vi "CreateReaderFromLib.vi"(0 "LibPath/LvLibRef":variant, 5 "error in":errorcluster) -> (14 "LibReader out":refnum<class "LibReader.lvclass">, 15 "Description":string, 16 "DataFlowClass":bool, 19 "error out":errorcluster)   [LabVIEW 2014, in "LibReader.lvclass"]
uses:
  <resource>/Framework/Providers/Open_GDS/ClassProviders/LibProvider_BaseClassInterface/LibReader_class/LibReader.lvclass
  <resource>/Framework/Providers/Open_GDS/ClassProviders/Provider_LvNativeClass/ClassReaderNative_class/ClassReaderNative.lvclass
  <resource>/Framework/Providers/Open_GDS/ClassProviders/Provider_EndevoGOOP300/ClassReaderGOOP300_class/ClassReaderGOOP300.lvclass
  <resource>/Framework/Providers/Open_GDS/ClassProviders/Provider_EndevoGOOP400/ClassReaderGOOP400_class/ClassReaderGOOP400.lvclass
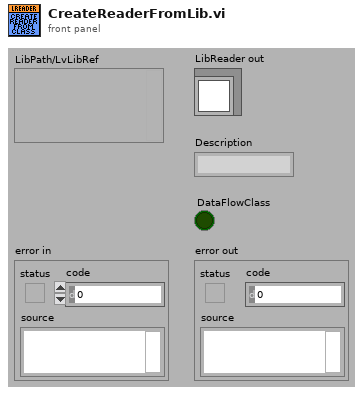
[diagram p1: front panel]
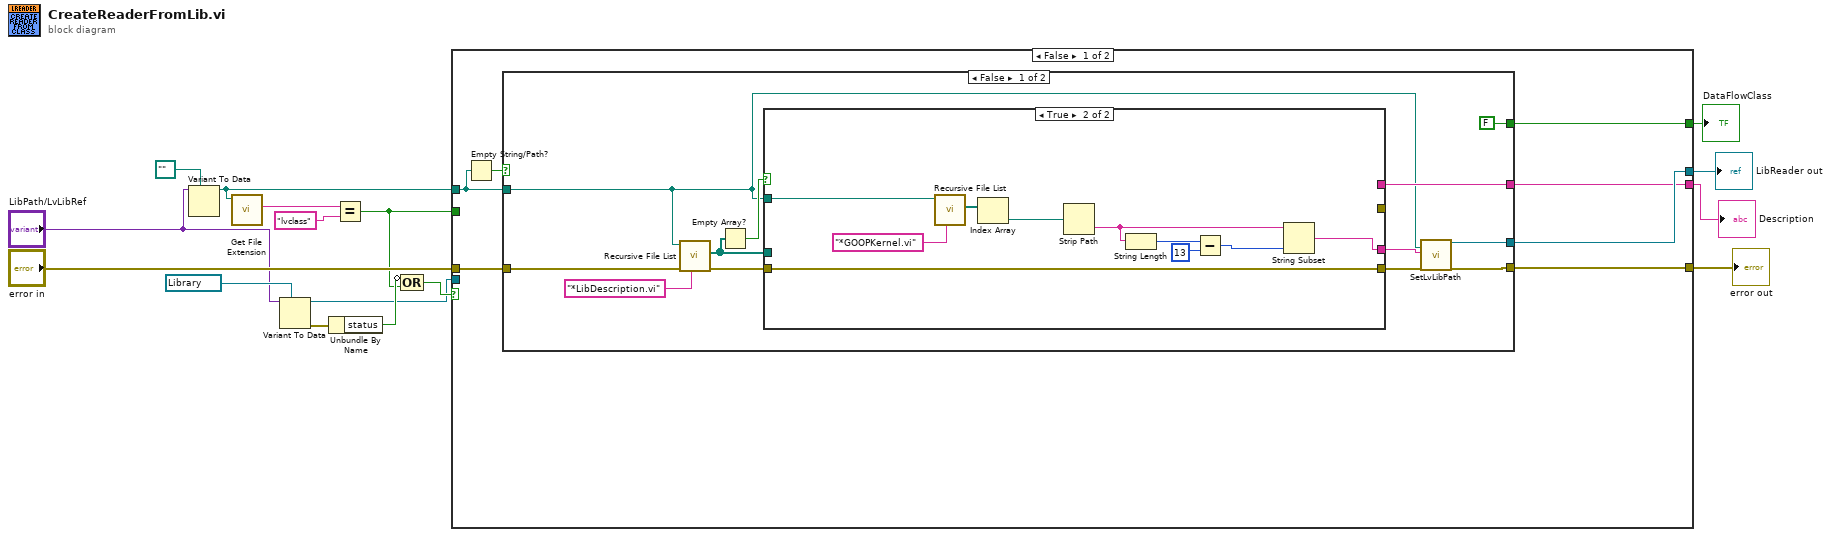
[diagram p0: block diagram]
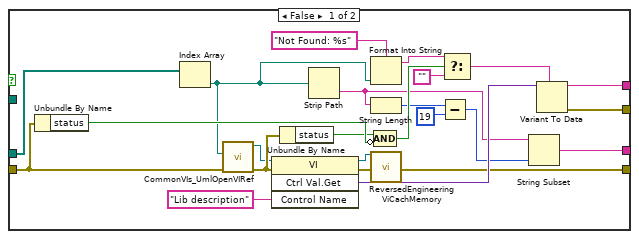
[diagram p2: hidden frame]
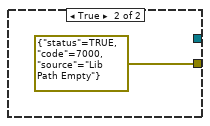
[diagram p3: hidden frame]
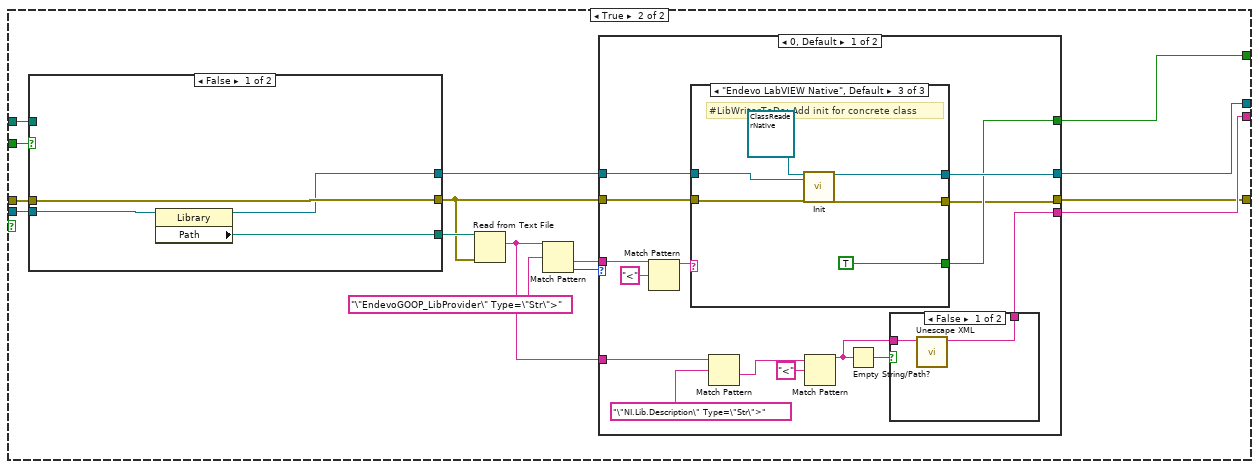
[diagram p4: hidden frame]
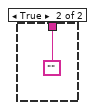
[diagram p5: hidden frame]
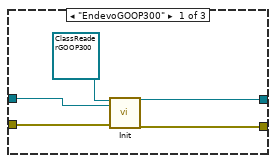
[diagram p6: hidden frame]
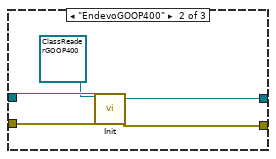
[diagram p7: hidden frame]
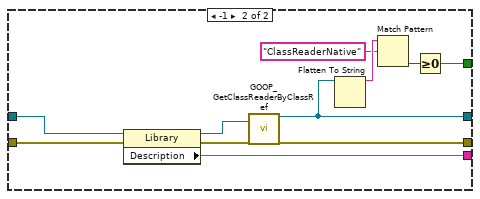
[diagram p8: hidden frame]
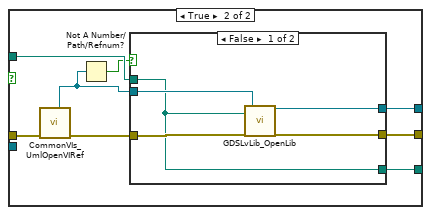
[diagram p9: hidden frame]
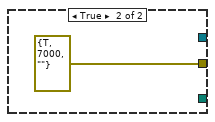
[diagram p10: hidden frame]
diagram:
  n1 = Variant To Data(type=path "", Variant="LibPath/LvLibRef") -> (data=w4:path)  [unwired: 1 in, 1 out]
  n2 = call <vilib>:"Get File Extension.vi"("file"=w4) -> ("lowercase file extension"=w9:string)  [unwired: 7 in, 3 out]
  n3 = Variant To Data(type=refnum<vi> refnum ("LVClass.Open"), Variant="LibPath/LvLibRef") -> (data=w3:refnum<vi>, error out=w7:errorcluster)  [unwired: 1 in]
  n4 = Unbundle By Name(w7) -> ("status"=w6:bool)
  n5 = Equal?(x=w9, y="lvclass") -> (x = y?=w2:bool)
  n6 = Compound Arithmetic op=OR(invert w6, w2) -> (w5:bool)
  n7 = case shown="False" w5 {
    tunnel: [w21 w85] -> w16
    tunnel: "error in" -> [w20 w83]
    tunnel: [w23 w78] -> w14
    tunnel: [w22 w82] -> w13
    tunnel: w4 -> [w18 w81]
    tunnel: w3 -> [_ w79]
    tunnel: w2 -> [_ w80]
    tunnel: [w19 w71] -> w1
    frame False {
      n8 = Empty String/Path?(string/path=w18) -> (empty?=w17:bool)
      n9 = case shown="False" w17 {
        tunnel: [w35 _] -> w23
        tunnel: [w34 errorcluster {"status"=TRUE, "code"=7000, "source"="Lib Path Empty"} ("error out")] -> w22
        tunnel: [w33 _] -> w21
        tunnel: w20 -> [w29 _]
        tunnel: [FALSE _] -> w19
        tunnel: w18 -> [w24 _]
        frame False {
          n10 = call <vilib>:"Recursive File List.vi"("pattern"="*LibDescription.vi" ("FileSearchPattern"), "error in (no error)"=w29, "Folder Path"=w24) -> ("error out"=w28:errorcluster, "All Files in Dir"=w26:path[])  [unwired: 4 in, 3 out]
          n11 = Empty Array?(array=w26) -> (empty?=w31:bool)
          n12 = case shown="True" w31 {
            tunnel: w28 -> [w45 w69]
            tunnel: [w50 _] -> w33
            tunnel: [w47 w69] -> w32
            tunnel: w26 -> [w46 _]
            tunnel: [w37 w60] -> w30
            tunnel: w24 -> [_ w68]
            tunnel: [w36 _] -> _
            frame False {
              n13 = Unbundle By Name(w45) -> ("status"=w52:bool)
              n14 = Index Array(array=w46) -> (element=w42:path)  [unwired: 1 in]
              n15 = call <resource>:"CommonVIs_UmlOpenVIRef.vi"("error in"=w45, "ViPath/ViName"=w42) -> ("error out"=w44:errorcluster, "vi reference"=w43:refnum<vi>)  [unwired: 6 in, 2 out]
              n16 = invoke class="VI" method="Ctrl Val.Get"(reference=w43, error in=w44, "Control Name"="Lib description") -> (reference out=w59:refnum<vi>, error out=w48:errorcluster, "Get Control Value Variant"=w58:variant)  [unwired: 1 in, 1 out]
              n17 = Unbundle By Name(w44) -> ("status"=w51:bool)
              n18 = Strip Path(path=w42) -> (name=w41:string)  [unwired: 1 out]
              n19 = Format Into String(format string="Not Found: %s", w42) -> (resulting string=w56:string)  [unwired: 2 in, 1 out]
              n20 = String Length(string=w41) -> (length=w40:i32)
              n21 = call <resource>:"ReversedEngineering ViCachMemory.vi"("ViRef"=w59, "error in (no error)"=w48) -> ("error out"=w47:errorcluster)  [unwired: 17 in]
              n22 = Compound Arithmetic op=AND(w51, invert w52) -> (w53:bool)
              n23 = Subtract(x=w40, y=19) -> (x-y=w39:i32)
              n24 = Select(t=w56, s=w53, f="") -> (s? t:f=w49:string)
              n25 = String Subset(string=w41, length (rest)=w39) -> (substring=w37:string)  [unwired: 1 in]
              n26 = Variant To Data(type=w49, Variant=w58) -> (data=w50:string, error out=w36:errorcluster)  [unwired: 1 in]
            }
            frame True {
              n27 = call <vilib>:"Recursive File List.vi"("pattern"="*GOOPKernel.vi", "Folder Path"=w68) -> ("All Files in Dir"=w62:path[])  [unwired: 5 in, 4 out]
              n28 = Index Array(array=w62) -> (element=w61:path)  [unwired: 1 in]
              n29 = Strip Path(path=w61) -> (name=w66:string)  [unwired: 1 out]
              n30 = String Length(string=w66) -> (length=w65:i32)
              n31 = Subtract(x=w65, y=13) -> (x-y=w64:i32)
              n32 = String Subset(string=w66, length (rest)=w64) -> (substring=w60:string)  [unwired: 1 in]
            }
          }
          n33 = call <resource>:"SetLvLibPath.vi"("LibPath"=w24, "LibName"=w30, "error in (no error)"=w32) -> ("LibReader out"=w35:refnum<class "LibReader.lvclass">, "error out"=w34:errorcluster)  [unwired: 15 in]
        }
        frame True {
        }
      }
    }
    frame True {
      n34 = case shown="False" w80 {
        tunnel: [w132 w136] -> w84
        tunnel: w83 -> [w134 w142]
        tunnel: [w134 w139] -> w76
        tunnel: w81 -> [_ w140]
        tunnel: w79 -> [w133 _]
        tunnel: [w131 w135] -> w77
        frame False {
          n35 = property class="Library"(reference=w133) -> (reference out=w132:refnum<vi>, "Path"=w131:path)  [unwired: 1 in, 1 out]
        }
        frame True {
          n36 = call <resource>:"CommonVIs_UmlOpenVIRef.vi"("error in"=w142) -> ("error out"=w141:errorcluster, "AppRefOut"=w137:refnum<vi>)  [unwired: 7 in, 2 out]
          n37 = Not A Number/Path/Refnum?(number/path/refnum=w137) -> (NaN/Path/Refnum?=w138:bool)
          n38 = case shown="False" w138 {
            tunnel: [w147 _] -> w136
            tunnel: w141 -> [w146 _]
            tunnel: w140 -> [w143 _]
            tunnel: [w145 errorcluster {"status"=TRUE, "code"=7000, "source"=""} ("error out")] -> w139
            tunnel: w137 -> [w144 _]
            tunnel: [w143 _] -> w135
            frame False {
              n39 = call <resource>:"GDSLvLib_OpenLib.vi"("LibToOpen"=w143, "error in (no error)"=w146, "Project/ApplicationRef(If empty, currect active project will be used)"=w144) -> ("LvLib"=w147:refnum<vi>, "error out"=w145:errorcluster)  [unwired: 15 in]
            }
            frame True {
            }
          }
        }
      }
      n40 = Read from Text File(file (use dialog)=w77, error in=w76) -> (text=w72:string)  [unwired: 2 in, 3 out]
      n41 = Match Pattern(string=w72, regular expression="\"EndevoGOOP_LibProvider\" Type=\"Str\">" ("y")) -> (after substring=w73:string, offset past match=w74:i32)  [unwired: 1 in, 2 out]
      n42 = case shown="0, Default" w74 {
        tunnel: [w91 w130] -> w85
        tunnel: w84 -> [w88 w129]
        tunnel: [w86 w128] -> w82
        tunnel: [w97 w121] -> w78
        tunnel: w76 -> [w87 w125]
        tunnel: w73 -> [w100 _]
        tunnel: w72 -> [w96 _]
        tunnel: [w89 w120] -> w71
        frame 0, Default {
          n43 = Match Pattern(string=w100, regular expression="<") -> (before substring=w98:string)  [unwired: 1 in, 3 out]
          n44 = case shown="\"Endevo LabVIEW Native\", Default" w98 {
            tunnel: [w108 w110 w118] -> w97
            tunnel: [_ _ TRUE] -> w89
            tunnel: w88 -> [w105 w112 w117]
            tunnel: w87 -> [w107 w113 w115]
            tunnel: [w106 w111 w116] -> w86
            frame "EndevoGOOP300" {
              n45 = call-dynamic "Init.vi"("ClassReaderGOOP300 in"=refnum<class "ClassReaderGOOP300.lvclass"> refnum, "LvClassRef"=w105, "error in (no error)"=w107) -> ("ClassReaderGOOP300 out"=w108:refnum<class "ClassReaderGOOP300.lvclass">, "error out"=w106:errorcluster)  [unwired: 15 in]
            }
            frame "EndevoGOOP400" {
              n46 = call-dynamic "Init.vi"("ClassReaderGOOP300 in"=refnum<class "ClassReaderGOOP400.lvclass"> refnum, "LvClassRef"=w112, "error in (no error)"=w113) -> ("ClassReaderGOOP300 out"=w110:refnum<class "ClassReaderGOOP400.lvclass">, "error out"=w111:errorcluster)  [unwired: 15 in]
            }
            frame "Endevo LabVIEW Native", Default {
              # "#LibWriterToDo: Add init for concrete class"
              n47 = call-dynamic "Init.vi"("ClassReaderNative in"=refnum<class "ClassReaderNative.lvclass"> refnum, "LvClassRef"=w117, "error in (no error)"=w115) -> ("ClassReaderNative out"=w118:refnum<class "ClassReaderNative.lvclass">, "error out"=w116:errorcluster)  [unwired: 15 in]
            }
          }
          n48 = Match Pattern(string=w96, regular expression="\"NI.Lib.Description\" Type=\"Str\">" ("y")) -> (after substring=w93:string)  [unwired: 1 in, 3 out]
          n49 = Match Pattern(string=w93, regular expression="<") -> (before substring=w90:string)  [unwired: 1 in, 3 out]
          n50 = Empty String/Path?(string/path=w90) -> (empty?=w92:bool)
          n51 = case shown="False" w92 {
            tunnel: [w101 ""] -> w91
            tunnel: w90 -> [w102 _]
            frame False {
              n52 = call <vilib>:"Unescape XML.vi"("XML String In"=w102) -> ("XML String Out"=w101:string)  [unwired: 9 in, 1 out]
            }
            frame True {
            }
          }
        }
        frame -1 {
          n53 = property class="Library"(reference=w129, error in=w125) -> (reference out=w127:refnum<vi>, error out=w126:errorcluster, "Description"=w130:string)
          n54 = call <resource>:"GOOP_GetClassReaderByClassRef.vi"("LVClassLibrary Refnum"=w127, "error in (no error)"=w126) -> ("ClassReaderNative out"=w121:refnum<class "ClassReaderNative.lvclass">, "error out"=w128:errorcluster)  [unwired: 16 in]
          n55 = Flatten To String(anything=w121) -> (data string=w124:string)  [unwired: 3 in, 2 out]
          n56 = Match Pattern(string=w124, regular expression="ClassReaderNative") -> (offset past match=w122:i32)  [unwired: 1 in, 3 out]
          n57 = Greater Or Equal To 0?(x=w122) -> (x >= 0?=w120:bool)
        }
      }
    }
  }
  "Description" <- w16
  "LibReader out" <- w14
  "error out" <- w13
  "DataFlowClass" <- w1
